vi "sensor-scale-vi.vi"(0 "input variable":dbl, 1 "v_max":dbl=3.3, 2 "param_max":dbl, 5 "V_0":dbl=1.52, 7 "param_0":dbl, 9 "V_1":dbl=1.56, 11 "param_1":dbl=1.176) -> (4 "output":dbl, 6 "output cluster":cluster{"current":dbl}, 8 "factor":dbl, 10 "offset":dbl, 15 "out_of_range_high":bool=TRUE)   [LabVIEW 2021]
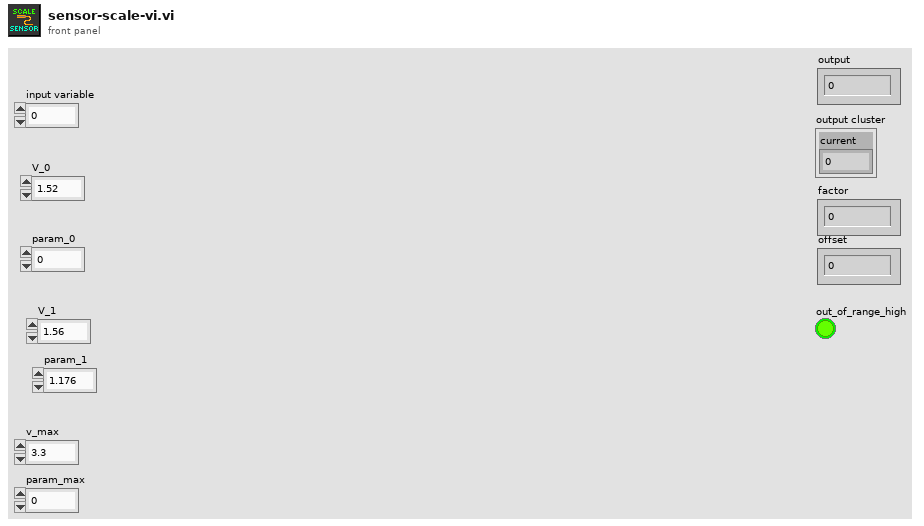
[diagram p1: front panel]
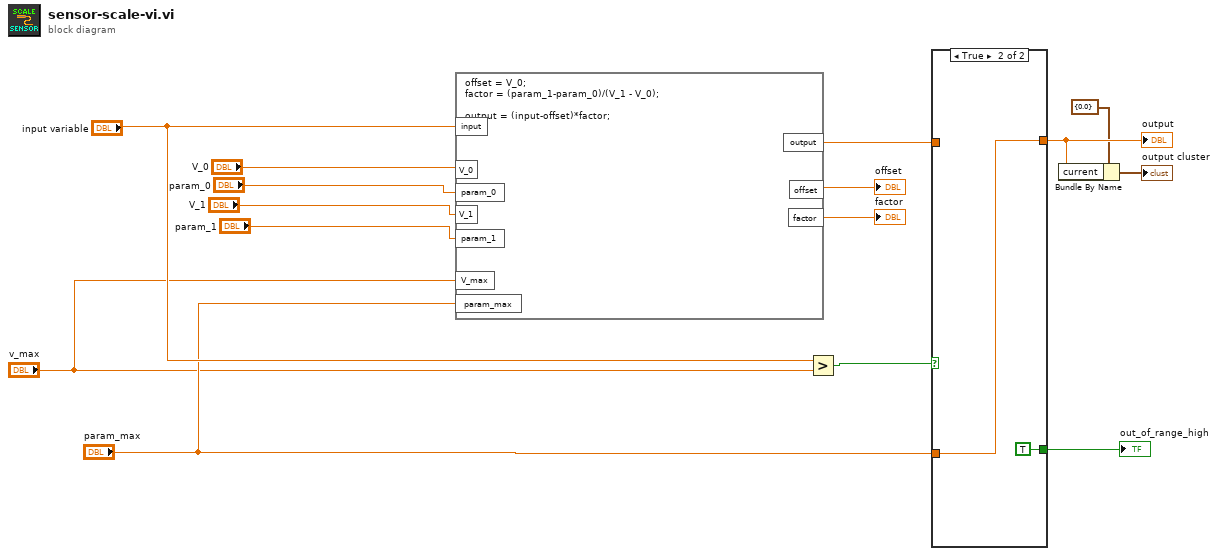
[diagram p0: block diagram]
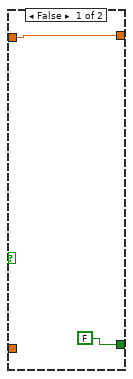
[diagram p2: hidden frame]
diagram:
  # "Set the range\nusing 2 points"
  n1 = formula code="offset = V_0;\nfactor = (param_1-param_0)/(V_1 - V_0);\n\noutput = (input-offset)*factor;"("V_0"="V_0", "V_1"="V_1", "param_0"="param_0", "param_1"="param_1", "input"="input variable", "V_max"="v_max", "param_max"="param_max") -> ("offset"=→"offset":dbl, "factor"=→"factor":dbl, "output"=w11:dbl)
  n2 = Greater?(x="input variable", y="v_max") -> (0:w12:bool)
  n3 = case shown="True" w12 {
    tunnel: w11 -> [w17 _]
    tunnel: [w17 w19] -> w3
    tunnel: "param_max" -> [_ w19]
    tunnel: [FALSE TRUE] -> w4
    frame False {
    }
    frame True {
    }
  }
  "output" <- w3
  "out_of_range_high" <- w4
  n4 = Bundle By Name(cluster=cluster{"current":dbl} {"current"=0.0} ("output cluster"), "current"=w3) -> (→"output cluster":cluster{"current":dbl})
